vi "DSCServer.vi"() -> ()   [LabVIEW 2010]
uses:
  Ctrls/ConnectStatus.ctl
  Ctrls/DeviceModel.ctl
  Drivers/ModbusServer/Serial Config.ctl
  Drivers/ModbusServer/DeviceListChannelData.ctl
  Drivers/ModbusServer/AutoChannelData.ctl
  Ctrls/ServerData.ctl
  Ctrls/DeviceInfomation.ctl
  Ctrls/ChannelData.ctl
  Ctrls/ChannelType.ctl
  Ctrls/ChannelAccessType.ctl
  Drivers/ModbusServer/DeviceListModbusAddressRegister.ctl
  Drivers/ModbusServer/ModbusAddressRegister.ctl
  Drivers/ModbusServer/MonitorServer.lvlib
panel:
  out "连接状态":T1[](array[typedef])
  in  "驱动配置":enum32{"WatlowF4", "CM51", "DCP551", "DPR250"}(tab)
  in  "F4配置":enum32{"设备配置", "变量查看"}(tab)
  in  "DeviceList":T3[](array[typedef])
  in  "ConfigModbus":bool
  out "AllRegisterData":i16[][](array[numeric])
  out "DeviceList":string[](array[string])
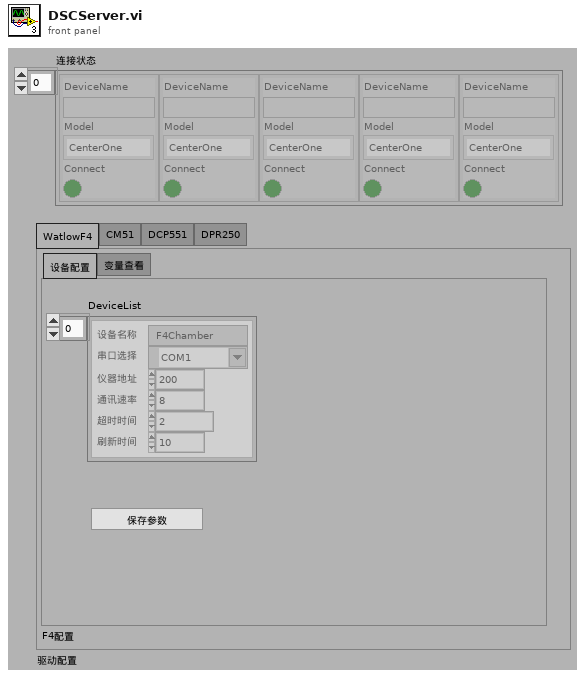
[diagram p1: front panel]
types:
  T1 = typedef "ConnectStatus.ctl" = cluster{"DeviceName":string, "Model":T2, "Connect":bool}
  T2 = typedef "DeviceModel.ctl" = enum16{"WatlowF4", "CenterOne", "DCP551", "DPR250"}
  T3 = typedef "MonitorServer.lvlib/Serial Config.ctl" = cluster{"设备名称":string, "串口选择":refnum<visa-resource-name>, "仪器地址":u32, "通讯速率":u32, "超时时间":u32, "刷新时间":dbl}
  T4 = enum32{"invalid app kind", "Development System", "Run Time System", "Student Edition", "Embedded LabVIEW", "Evaluation", "Custom"}
  T5 = enum32{"Invalid", "Standard", "Closed", "Hidden", "Minimized", "Maximized"}
  T6 = cluster{"Core":cluster{"Current VI Reference":refnum<vi>, "Close Panel on Exit?":bool}, "Your Boolean data":bool, "Your string data":string}
  T7 = cluster{"Current VI Reference":refnum<vi>, "Close Panel on Exit?":bool}
  T8 = typedef "MonitorServer.lvlib/DeviceListChannelData.ctl" = T9[]
  T9 = typedef "MonitorServer.lvlib/AutoChannelData.ctl" = cluster{"DeviceName":string, "Channel1":dbl, "SetPoint1":dbl, "Channel2":dbl, "SetPoint2":dbl, "ConnectOK":bool, "DecimalPoint1":i16, "DecimalPoint2":i16}
  T10 = typedef "MonitorServer.lvlib/DeviceListModbusAddressRegister.ctl" = T11[]
  T11 = typedef "MonitorServer.lvlib/ModbusAddressRegister.ctl" = cluster{"DeviceName":string, "AllRegisterData":i16[]}
  T12 = typedef "ServerData.ctl" = T13[]
  T13 = typedef "DeviceInfomation.ctl" = cluster{"Model":T2, "ChamberName":string, "ChannelNumber":i32, "ChannelsData":T14[], "Connected":bool}
  T14 = typedef "ChannelData.ctl" = cluster{"ChannelName":string, "ChannelType":T15, "AccessType":T16, "ProcessValue":dbl, "SetValue":dbl, "NewSettValue":dbl, "SetNewTarget":bool}
  T15 = typedef "ChannelType.ctl" = enum16{"Temperature", "Humidity"}
  T16 = typedef "ChannelAccessType.ctl" = enum16{"ReadOnly", "SetTarget"}
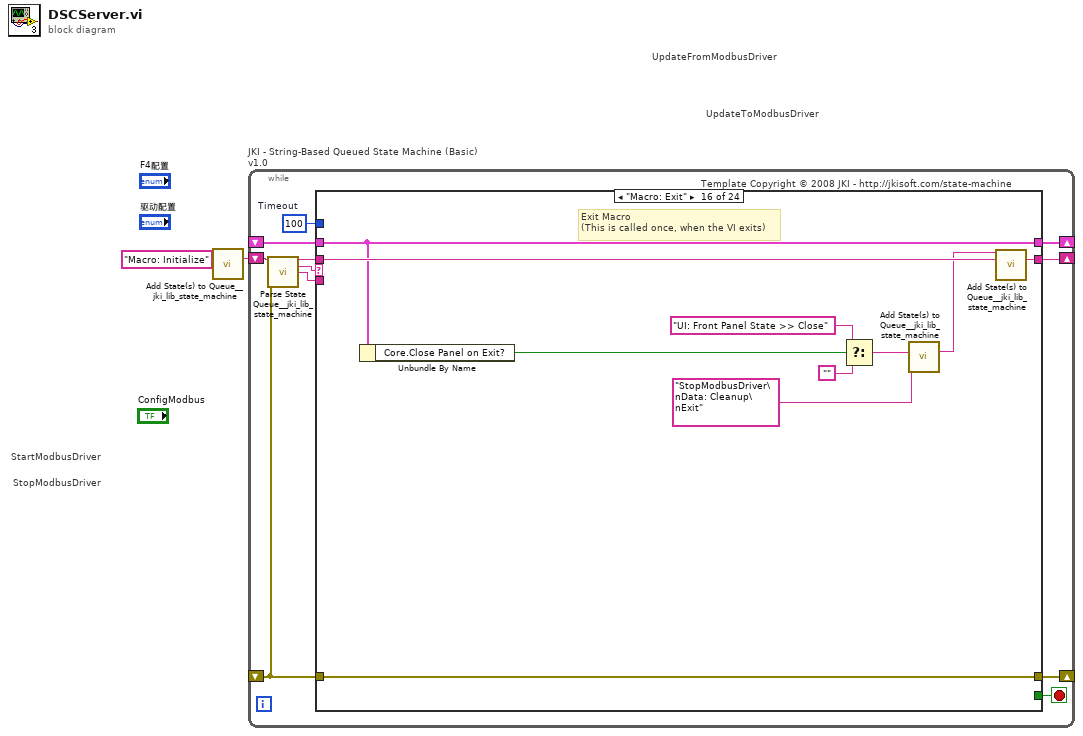
[diagram p0: block diagram]
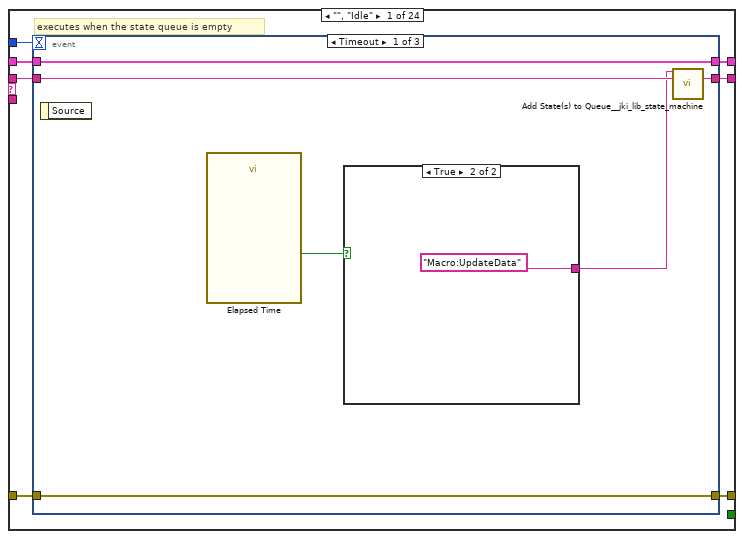
[diagram p2: hidden frame]
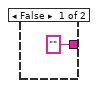
[diagram p3: hidden frame]
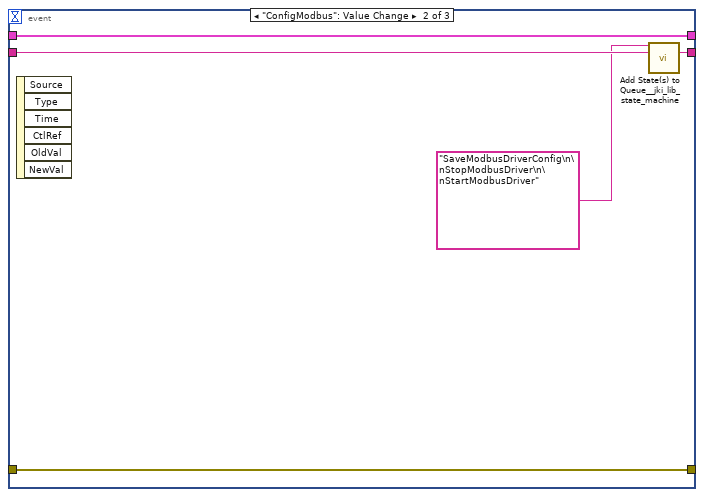
[diagram p4: hidden frame]
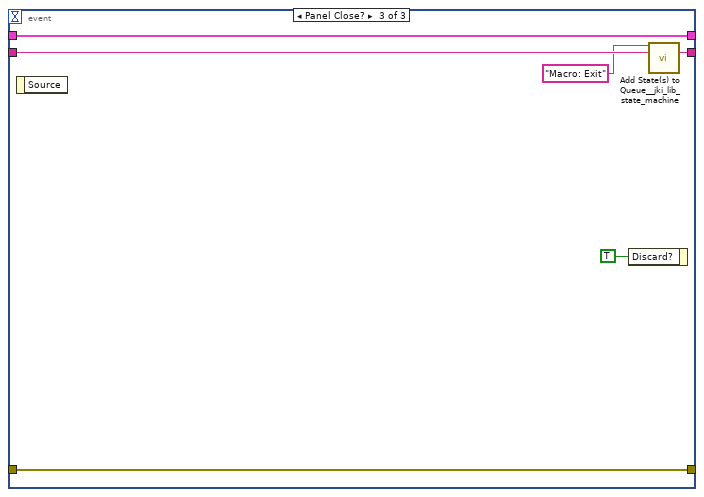
[diagram p5: hidden frame]
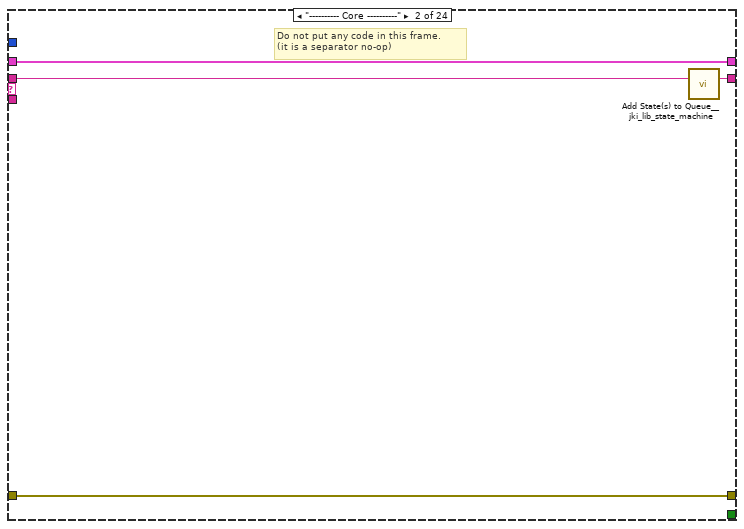
[diagram p6: hidden frame]
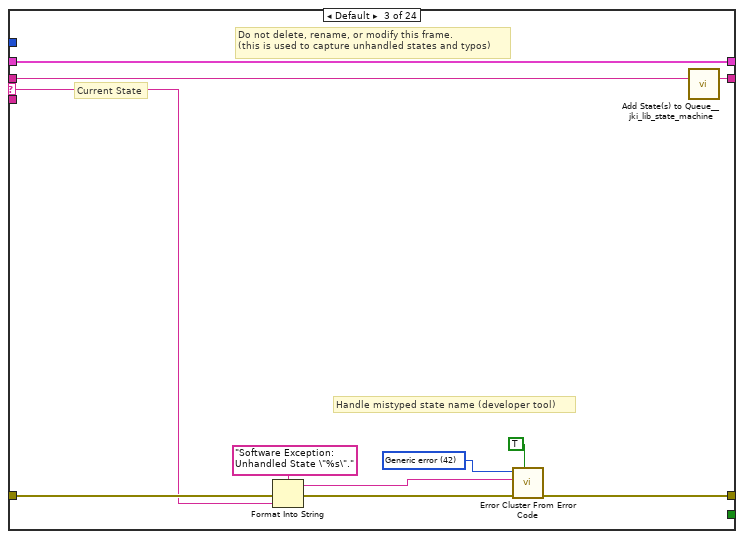
[diagram p7: hidden frame]
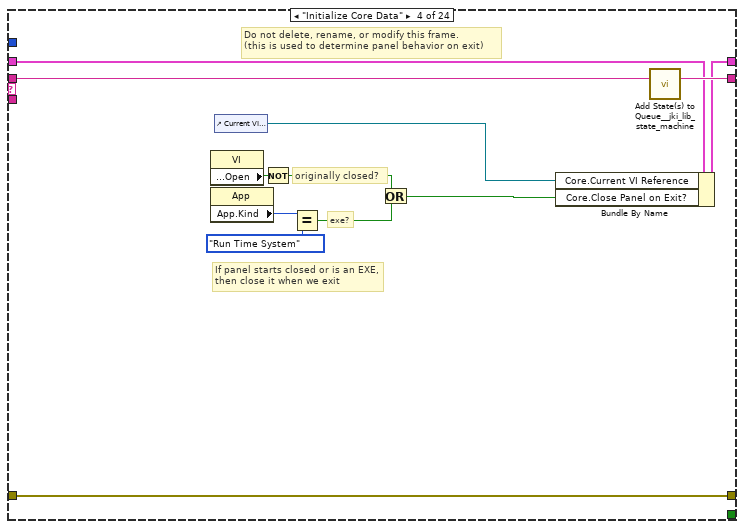
[diagram p8: hidden frame]
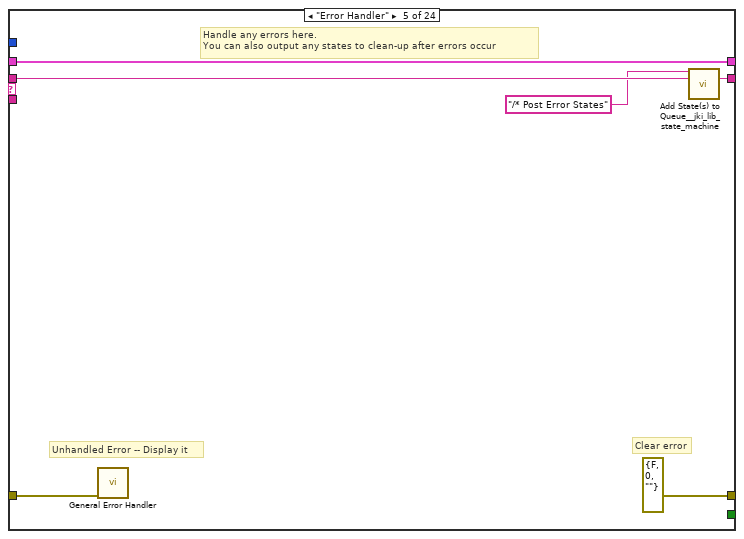
[diagram p9: hidden frame]
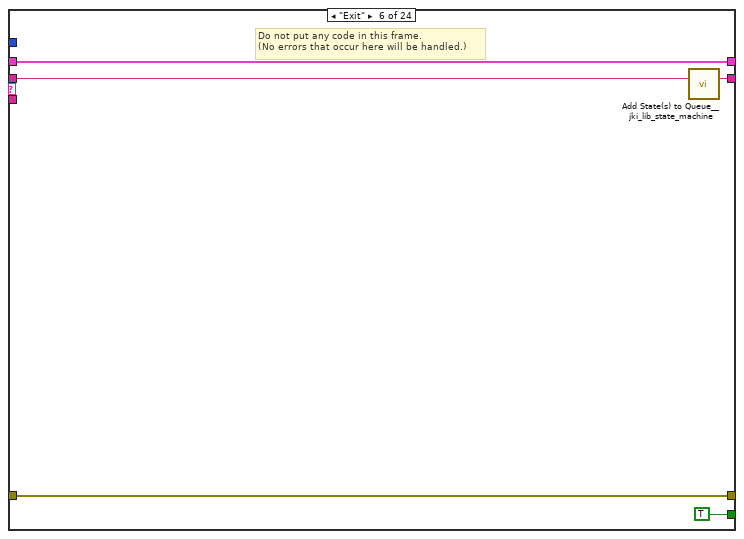
[diagram p10: hidden frame]
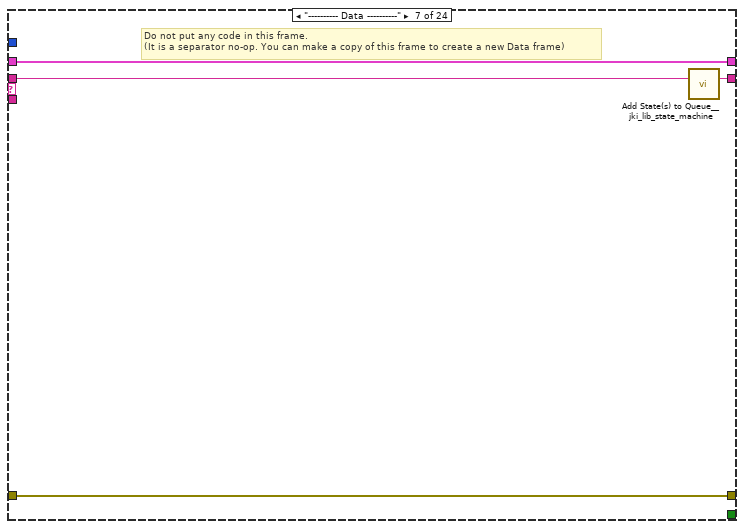
[diagram p11: hidden frame]
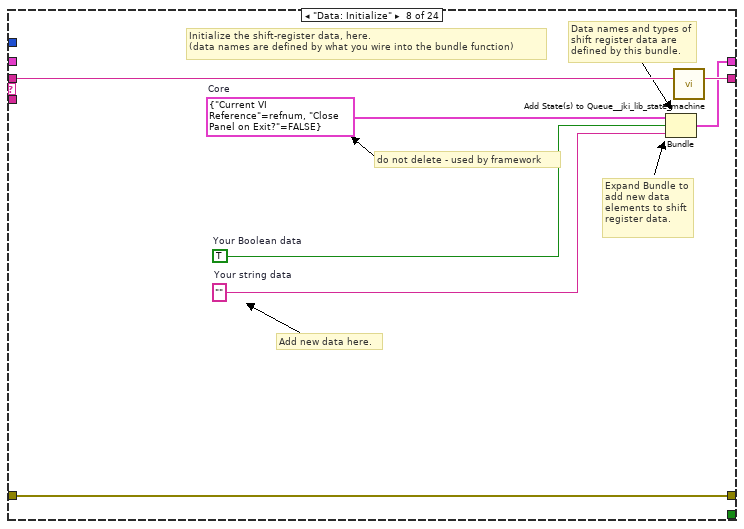
[diagram p12: hidden frame]
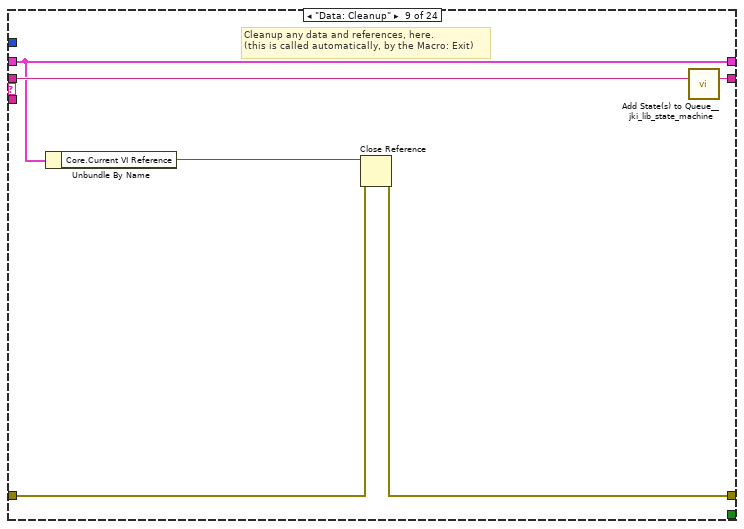
[diagram p13: hidden frame]
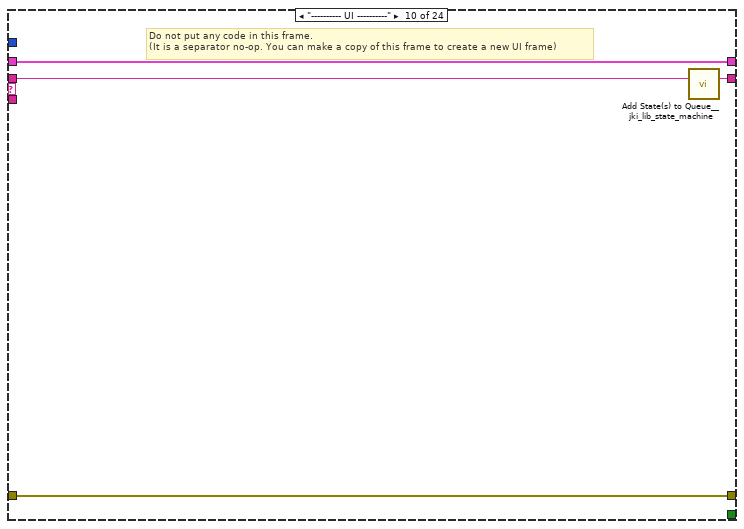
[diagram p14: hidden frame]
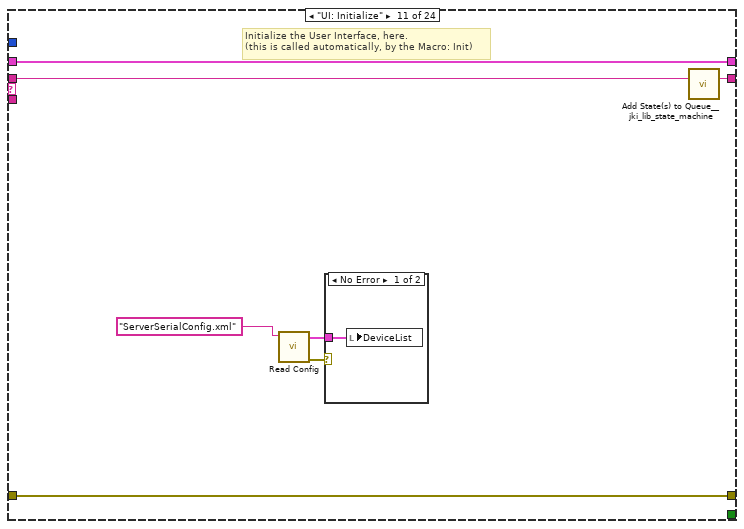
[diagram p15: hidden frame]
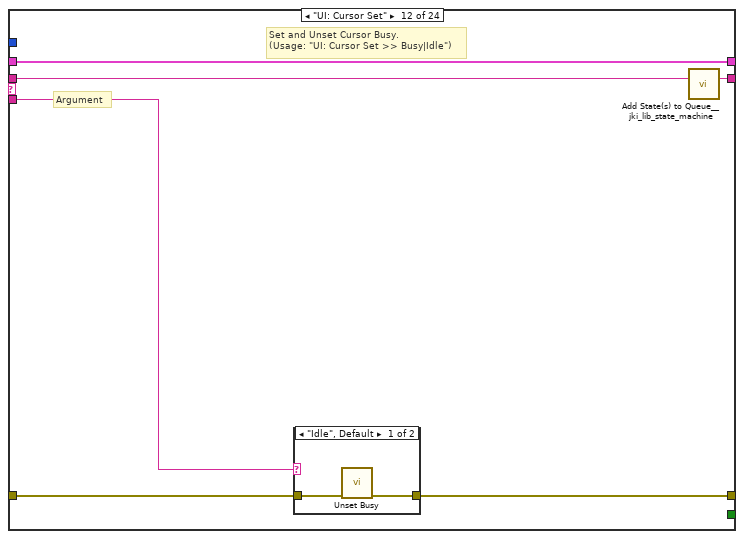
[diagram p17: hidden frame]
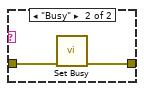
[diagram p18: hidden frame]
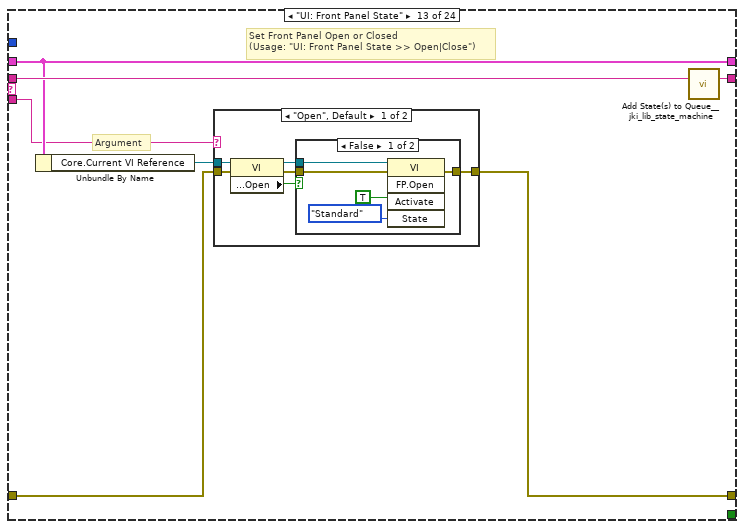
[diagram p19: hidden frame]
diagram:
  # "StopModbusDriver"
  # "StartModbusDriver"
  # "UpdateToModbusDriver"
  # "UpdateFromModbusDriver"
  n1 = call "Add State(s) to Queue__jki_lib_state_machine.vi"("State(s) in (\"\")"="Macro: Initialize") -> ("States Out"=w1:string)  [unwired: 14 in]
  n2 = while "JKI - String-Based Queued State Machine (Basic) v1.0" {
    shift-right: [w6] -> _
    shift-left: _ -> [w5]
    shift-right: [w9] -> _
    shift-left: _ -> [w3]
    shift-right: [w8] -> _
    shift-left: w1 -> [w10]
    stop <- w7 stop-if-true
    w4 = 100  # Timeout
    # "Template Copyright © 2008 JKI - http://jkisoft.com/state-machine"
    n3 = call "Parse State Queue__jki_lib_state_machine.vi"("State Queue"=w10, "Error In (no error)"=w3) -> ("Remaining States"=w12:string, "Current State"=w13:string, "Arguments"=w11:string)  [unwired: 11 in]
    n4 = case shown="\"Macro: Exit\"" w13 {
      selector: w13 -> [_ _ w44 _ _ _ _ _ _ _ _ _ _ _ _ _ _ _ _ _ _ _ _ _]
      tunnel: w12 -> [w20 w43 w48 w66 w72 w77 w81 w88 w94 w98 w105 w112 w123 w149 w154 w164 w169 w173 w179 w183 w187 w197 w206 w210]
      tunnel: w11 -> [_ _ _ _ _ _ _ _ _ _ _ w107 w117 _ _ _ _ _ _ _ _ _ _ _]
      tunnel: w5 -> [w18 w40 w46 w57 w69 w75 w78 _ w89 w95 w103 w110 w119 w146 w151 w161 w166 w170 w176 w180 w184 w194 w203 w207]
      tunnel: [w17 w41 w50 w63 errorcluster {"status"=FALSE, "code"=0, "source"=""} ("error out") w74 w79 w85 w90 w96 w102 w108 w120 w147 w152 w162 w167 w171 w177 w181 w185 w195 w204 w208] -> w9
      tunnel: w3 -> [w16 w41 w49 w63 w68 w74 w79 w85 w91 w96 w102 w109 w121 w147 w152 w162 w167 w171 w177 w181 w185 w195 w204 w208]
      tunnel: [w19 w42 w47 w65 w71 w76 w80 w87 w93 w97 w104 w111 w122 w148 w153 w163 w168 w172 w178 w182 w186 w196 w205 w209] -> w8
      tunnel: [_ _ _ _ _ TRUE _ _ _ _ _ _ _ _ _ _ _ _ _ _ _ _ _ _] -> w7
      tunnel: [w15 w40 w46 w64 w69 w75 w78 w86 w89 w95 w103 w110 w119 w146 w151 w161 w166 w170 w176 w180 w184 w194 w203 w207] -> w6
      tunnel: w4 -> [w14 _ _ _ _ _ _ _ _ _ _ _ _ _ _ _ _ _ _ _ _ _ _ _]
      frame "", "Idle" {
        # "executes when the state queue is empty"
        n5 = event shown="[0] Timeout" {
          selector: _ -> [_ _ _]
          dyn-events: _ -> [_ _ _]
          timeout: w14 -> [_ _ _]
          tunnel: w20 -> [w26 w33 w39]
          tunnel: [w25 w32 w38] -> w19
          tunnel: w18 -> [w23 w30 w36]
          tunnel: [w24 w31 w37] -> w17
          tunnel: w16 -> [w24 w31 w37]
          tunnel: [w23 w30 w36] -> w15
          event Timeout {
            n6 = event-data() -> ()  [unwired: 1 in, 1 out]
            n7 = call "Elapsed Time"() -> ("Time has Elapsed"=w22:bool)  [unwired: 12 in, 7 out]
            n8 = case shown="True" w22 {
              tunnel: ["" ("State(s) in Front (\"\")") "Macro:UpdateData" ("State(s) in Front (\"\")")] -> w21
              frame False {
              }
              frame True {
              }
            }
            n9 = call "Add State(s) to Queue__jki_lib_state_machine.vi"("State(s) in Front (\"\")"=w21, "State(s) in (\"\")"=w26) -> ("States Out"=w25:string)  [unwired: 13 in]
          }
          event "ConfigModbus": Value Change {
            n10 = event-data() -> ()  [unwired: 1 in, 6 out]
            n11 = call "Add State(s) to Queue__jki_lib_state_machine.vi"("State(s) in Front (\"\")"="SaveModbusDriverConfig\n\nStopModbusDriver\n\nStartModbusDriver" ("State(s) in Front (\"\")"), "State(s) in (\"\")"=w33) -> ("States Out"=w32:string)  [unwired: 13 in]
          }
          event Panel Close? {
            n12 = event-data() -> ()  [unwired: 1 in, 1 out]
            n13 = event-data("Discard?"=TRUE) -> ()  [unwired: 1 in, 1 out]
            n14 = call "Add State(s) to Queue__jki_lib_state_machine.vi"("State(s) in Front (\"\")"="Macro: Exit", "State(s) in (\"\")"=w39) -> ("States Out"=w38:string)  [unwired: 13 in]
          }
        }
      }
      frame "---------- Core ----------" {
        # "Do not put any code in this frame.\n(it is a separator no-op)"
        n15 = call "Add State(s) to Queue__jki_lib_state_machine.vi"("State(s) in (\"\")"=w43) -> ("States Out"=w42:string)  [unwired: 14 in]
      }
      frame Default {
        w53 = 42 items=["No error", "Argument error", "Memory is full", "Out of zone", "End of file", "File already open", "Generic file I/O error", "File not found", "File permission error", "Disk is full", "Duplicate path", "Too many files open", "System feature not enabled", "Resource file not found", "Cannot add resource", "Resource not found", "Image not found", "Image memory error", "Pen does not exist", "Config type invalid", "Config token not found", "Config parse error", "Config memory error", "Bad external code format", "Bad external code offset", "External code not present", "Null window", "Destroy window error", "Null menu", "Print aborted", "Bad print record", "Print driver error", "Windows error during printing", "Memory error during printing", "Print dialog error", "Generic print error", "Invalid device refnum", "Device not found", "Device parameter error", "Device unit error", "Cannot open device", "Device call aborted", "Generic error", "Cancelled by user", "Object ID too low", "Object ID too high", "Object not in heap", "Unknown heap", "Unknown object (invalid DefProc)", "Unknown object (DefProc not in table)", "Message out of range", "Invalid (null) method", "Unknown message", "Manager call not supported", "Bad address", "Network operation in progress", "Network operation timed out", "Connection is busy", "Network attribute not supported", "Network error", "Address in use", "System out of memory", "Connection aborted", "Connection refused", "Not connected", "Already connected", "Connection closed", "Initialization error (interapplication manager)", "Bad occurrence", "Wait on unbound occurrence handler", "Occurrence queue overflow", "Datalog type conflict", "Unused", "Unrecognized type (interapplication manager)", "Memory corrupt", "Failed to make temporary DLL", "Old CIN version", "Drag socket not found", "Failed to load drop-object", "Failed to register OLE object", "Failed to release OLE object", "Format specifier type mismatch", "Unknown format specifier", "Too few format specifiers", "Too many format specifiers", "Scan failed", "Newer CIN version", "Error converting to variant", "Runtime menu error", "Password tampered", "Variant attribute not found", "Incompatible variant data type", "Event data is not available", "Event Store is not present", "Occurrence is not found", "Event Queue is not created", "Event info is not available", "Refnum passed is NULL", "Error retrieving Class GUID", "Error retrieving CoClass GUID", "Error retrieving TypeLib GUID.", "Bad built application magic bytes.", "Specific driver is different from the specific driver associated with the Logical Name.", "There is no session opened to the class driver.", "Max Error", "MAX - Error with config objects", "MAX - Error loading configuration", "MAX - Group not supported"]
        # "Current State"
        # "Do not delete, rename, or modify this frame.\n(this is used to capture unhandled states and typos)"
        # "Handle mistyped state name (developer tool)"
        n16 = Format Into String(format string="Software Exception: Unhandled State \"%s\"." ("message"), error in=w49, w44) -> (resulting string=w52:string, error out=w51:errorcluster)  [unwired: 1 in]
        n17 = call <vilib>:"Error Cluster From Error Code.vi"("show call chain? (False)"=TRUE, "error in (no error)"=w51, "error message (\"\")"=w52, "error code (0)"=w53) -> ("error out"=w50:errorcluster)  [unwired: 5 in]
        n18 = call "Add State(s) to Queue__jki_lib_state_machine.vi"("State(s) in (\"\")"=w48) -> ("States Out"=w47:string)  [unwired: 14 in]
      }
      frame "Initialize Core Data" {
        # "Do not delete, rename, or modify this frame.\n(this is used to determine panel behavior on exit)"
        # "originally closed?"
        # "exe?"
        # "If panel starts closed or is an EXE, then close it when we exit"
        n19 = property class="VI"() -> ("Front Panel.Open"=w62:bool)  [unwired: 2 in, 2 out]
        n20 = property class="App"() -> ("App.Kind"=w61:T4)  [unwired: 2 in, 2 out]
        n21 = control-ref of="Current VI Reference"() -> (w55:refnum<vi>)
        n22 = Not(x=w62) -> (.not. x?=w59:bool)
        n23 = Equal?(x=w61, y=T4."Run Time System" ("Application:Kind")) -> (x = y?=w58:bool)
        n24 = Or(x=w59, y=w58) -> (x .or. y?=w56:bool)
        n25 = Bundle By Name(cluster=w57, "Core.Current VI Reference"=w55, "Core.Close Panel on Exit?"=w56) -> (w64:T6)
        n26 = call "Add State(s) to Queue__jki_lib_state_machine.vi"("State(s) in (\"\")"=w66) -> ("States Out"=w65:string)  [unwired: 14 in]
      }
      frame "Error Handler" {
        # "Unhandled Error -- Display it"
        # "Handle any errors here.\nYou can also output any states to clean-up after errors occur"
        # "Clear error"
        n27 = call <vilib>:"General Error Handler.vi"("error in (no error)"=w68) -> ()  [unwired: 10 in, 5 out]
        n28 = call "Add State(s) to Queue__jki_lib_state_machine.vi"("State(s) in Front (\"\")"="/* Post Error States", "State(s) in (\"\")"=w72) -> ("States Out"=w71:string)  [unwired: 13 in]
      }
      frame "Exit" {
        # "Do not put any code in this frame.\n(No errors that occur here will be handled.)"
        n29 = call "Add State(s) to Queue__jki_lib_state_machine.vi"("State(s) in (\"\")"=w77) -> ("States Out"=w76:string)  [unwired: 14 in]
      }
      frame "---------- Data ----------" {
        # "Do not put any code in this frame.\n(It is a separator no-op. You can make a copy of this frame to create a new Data frame)"
        n30 = call "Add State(s) to Queue__jki_lib_state_machine.vi"("State(s) in (\"\")"=w81) -> ("States Out"=w80:string)  [unwired: 14 in]
      }
      frame "Data: Initialize" {
        w82 = T7 {"Current VI Reference"=refnum, "Close Panel on Exit?"=FALSE}  # Core
        w84 = TRUE  # Your Boolean data
        w83 = ""  # Your string data
        # "do not delete - used by framework"
        # "Expand Bundle to add new data elements to shift register data."
        # "Add new data here."
        # "Data names and types of shift register data are defined by this bundle."
        # "Initialize the shift-register data, here.\n(data names are defined by what you wire into the bundle function)"
        n31 = Bundle("Core"=w82, "Your Boolean data"=w84, "Your string data"=w83) -> (w86:T6)  [unwired: 1 in]
        n32 = call "Add State(s) to Queue__jki_lib_state_machine.vi"("State(s) in (\"\")"=w88) -> ("States Out"=w87:string)  [unwired: 14 in]
      }
      frame "Data: Cleanup" {
        # "Cleanup any data and references, here.\n(this is called automatically, by the Macro: Exit)"
        n33 = Unbundle By Name(w89) -> ("Core.Current VI Reference"=w92:refnum<vi>)
        n34 = Close Reference(reference=w92, error in (no error)=w91) -> (error out=w90:errorcluster)
        n35 = call "Add State(s) to Queue__jki_lib_state_machine.vi"("State(s) in (\"\")"=w94) -> ("States Out"=w93:string)  [unwired: 14 in]
      }
      frame "---------- UI ----------" {
        # "Do not put any code in this frame.\n(It is a separator no-op. You can make a copy of this frame to create a new UI frame)"
        n36 = call "Add State(s) to Queue__jki_lib_state_machine.vi"("State(s) in (\"\")"=w98) -> ("States Out"=w97:string)  [unwired: 14 in]
      }
      frame "UI: Initialize" {
        # "Initialize the User Interface, here.\n(this is called automatically, by the Macro: Init)"
        n37 = call "Read Config.vi"("ConfigurationFileName"="ServerSerialConfig.xml" ("FileName")) -> ("error out"=w99:errorcluster, "DeviceList"=w100:T3[])  [unwired: 9 in]
        n38 = case shown="No Error" w99 {
          tunnel: w100 -> [w106 _]
          frame No Error {
            n39 = local write "DeviceList"(w106) -> ()
          }
          frame Error {
          }
        }
        n40 = call "Add State(s) to Queue__jki_lib_state_machine.vi"("State(s) in (\"\")"=w105) -> ("States Out"=w104:string)  [unwired: 14 in]
      }
      frame "UI: Cursor Set" {
        # "Argument"
        # "Set and Unset Cursor Busy.\n(Usage: \"UI: Cursor Set >> Busy|Idle\")"
        n41 = case shown="\"Idle\", Default" w107 {
          tunnel: w109 -> [w114 w116]
          tunnel: [w113 w115] -> w108
          frame "Idle", Default {
            n42 = call <vilib>:"Unset Busy.vi"("error in (no error)"=w114) -> ("error out"=w113:errorcluster)  [unwired: 10 in]
          }
          frame "Busy" {
            n43 = call <vilib>:"Set Busy.vi"("error in (no error)"=w116) -> ("error out"=w115:errorcluster)  [unwired: 9 in, 1 out]
          }
        }
        n44 = call "Add State(s) to Queue__jki_lib_state_machine.vi"("State(s) in (\"\")"=w112) -> ("States Out"=w111:string)  [unwired: 14 in]
      }
      frame "UI: Front Panel State" {
        # "Argument"
        # "Set Front Panel Open or Closed\n(Usage: \"UI: Front Panel State >> Open|Close\")"
        n45 = Unbundle By Name(w119) -> ("Core.Current VI Reference"=w118:refnum<vi>)
        n46 = case shown="\"Open\", Default" w117 {
          tunnel: w121 -> [w127 w140]
          tunnel: [w129 w141] -> w120
          tunnel: w118 -> [w128 w138]
          frame "Open", Default {
            n47 = property class="VI"(reference=w128, error in=w127) -> (reference out=w125:refnum<vi>, error out=w126:errorcluster, "Front Panel.Open"=w124:bool)
            n48 = case shown="False" w124 {
              tunnel: [w132 w135] -> w129
              tunnel: w126 -> [w131 w135]
              tunnel: w125 -> [w130 _]
              frame False {
                n49 = invoke class="VI" method="FP.Open"(reference=w130, error in=w131, "Activate"=TRUE, "State"=T5."Standard") -> (error out=w132:errorcluster)  [unwired: 1 in, 4 out]
              }
              frame True {
              }
            }
          }
          frame "Close" {
            n50 = property class="VI"(reference=w138, error in=w140) -> (reference out=w137:refnum<vi>, error out=w139:errorcluster, "Front Panel.Open"=w136:bool)
            n51 = case shown="True" w136 {
              tunnel: [w142 w145] -> w141
              tunnel: w139 -> [w142 w144]
              tunnel: w137 -> [_ w143]
              frame False {
              }
              frame True {
                n52 = invoke class="VI" method="FP.Close"(reference=w143, error in=w144) -> (error out=w145:errorcluster)  [unwired: 1 in, 2 out]
              }
            }
          }
        }
        n53 = call "Add State(s) to Queue__jki_lib_state_machine.vi"("State(s) in (\"\")"=w123) -> ("States Out"=w122:string)  [unwired: 14 in]
      }
      frame "---------- Macro ----------" {
        # "Do not put any code in this frame.\n(It is a separator no-op. You can make a copy of this frame to create a new Macro frame)"
        n54 = call "Add State(s) to Queue__jki_lib_state_machine.vi"("State(s) in (\"\")"=w149) -> ("States Out"=w148:string)  [unwired: 14 in]
      }
      frame "Macro: Initialize" {
        w150 = "Data: Initialize\nInitialize Core Data\nUI: Initialize\nUI: Front Panel State >> Open\nStartModbusDriver\n"  # Data: Initialize Initialize Core Data UI: Initialize UI: Front Panel State >> Open StartModbusDriver
        # "Initialization Macro\n(This is called once, when the VI starts)"
        n55 = call "Add State(s) to Queue__jki_lib_state_machine.vi"("State(s) in Front (\"\")"=w150, "State(s) in (\"\")"=w154) -> ("States Out"=w153:string)  [unwired: 13 in]
      }
      frame "Macro: Exit" {
        # "Exit Macro\n(This is called once, when the VI exits)"
        n56 = Unbundle By Name(w161) -> ("Core.Close Panel on Exit?"=w160:bool)
        n57 = Select(t="UI: Front Panel State >> Close", s=w160, f="") -> (s? t:f=w157:string)
        n58 = call "Add State(s) to Queue__jki_lib_state_machine.vi"("State(s) in (\"\")"=w157, "State(s) at Back (\"\")"="StopModbusDriver\nData: Cleanup\nExit") -> ("States Out"=w155:string)  [unwired: 13 in]
        n59 = call "Add State(s) to Queue__jki_lib_state_machine.vi"("State(s) in Front (\"\")"=w155, "State(s) in (\"\")"=w164) -> ("States Out"=w163:string)  [unwired: 13 in]
      }
      frame "Macro:UpdateData" {
        # "Exit Macro\n(This is called once, when the VI exits)"
        n60 = call "Add State(s) to Queue__jki_lib_state_machine.vi"("State(s) in Front (\"\")"="UpdateFromModbusDriver\nUpdateToModbusDriver" ("State(s) in Front (\"\")"), "State(s) in (\"\")"=w169) -> ("States Out"=w168:string)  [unwired: 13 in]
      }
      frame "---------- ModbusDriver ----------" {
        # "Template Separator\n(You can make a copy of, or modify, this frame)"
        n61 = call "Add State(s) to Queue__jki_lib_state_machine.vi"("State(s) in (\"\")"=w173) -> ("States Out"=w172:string)  [unwired: 14 in]
      }
      frame "SaveModbusDriverConfig" {
        # "Your code here.\n(You can make a copy of, or modify, this frame)"
        n62 = call "Save Config.vi"("FileName"="ServerSerialConfig.xml", "DeviceList"="DeviceList") -> ()  [unwired: 9 in, 1 out]
        n63 = call "Add State(s) to Queue__jki_lib_state_machine.vi"("State(s) in (\"\")"=w179) -> ("States Out"=w178:string)  [unwired: 14 in]
      }
      frame "StartModbusDriver" {
        # "Your code here.\n(You can make a copy of, or modify, this frame)"
        n64 = call "StartServer.vi"() -> ()  [unwired: 11 in, 1 out]
        n65 = call "Add State(s) to Queue__jki_lib_state_machine.vi"("State(s) in (\"\")"=w183) -> ("States Out"=w182:string)  [unwired: 14 in]
      }
      frame "StopModbusDriver" {
        # "Your code here.\n(You can make a copy of, or modify, this frame)"
        n66 = call "StopServer.vi"() -> ()  [unwired: 11 in, 1 out]
        n67 = call "Add State(s) to Queue__jki_lib_state_machine.vi"("State(s) in (\"\")"=w187) -> ("States Out"=w186:string)  [unwired: 14 in]
      }
      frame "UpdateFromModbusDriver" {
        n68 = shared-variable "My Computer\\MonitorServer.lvlib\\AutoReadChannels"() -> (w193:T8)  [unwired: 1 in, 1 out]
        n69 = shared-variable "My Computer\\MonitorServer.lvlib\\DeviceListRegister"() -> (w190:T10)  [unwired: 1 in, 1 out]
        n70 = for {
          tunnel: w190 -> [w200] mode=indexing
          tunnel: [w199] -> w188 mode=indexing
          tunnel: [w198] -> w189 mode=indexing
          n71 = Unbundle By Name(w200) -> ("DeviceName"=w199:string, "AllRegisterData"=w198:i16[])
        }
        "AllRegisterData" <- w189
        "DeviceList" <- w188
        n72 = call "ModbusDriverDataToServer.vi"("DeviceListChannelData"=w193) -> ("ServerData"=w192:T12, "Status"=→"连接状态":T1[])  [unwired: 9 in]
        n73 = shared-variable "My Computer\\DSCServer.lvlib\\ServerData"(w192) -> ()  [unwired: 1 in, 1 out]
        n74 = call "Add State(s) to Queue__jki_lib_state_machine.vi"("State(s) in (\"\")"=w197) -> ("States Out"=w196:string)  [unwired: 14 in]
      }
      frame "UpdateToModbusDriver" {
        n75 = shared-variable "My Computer\\MonitorServer.lvlib\\AutoReadChannels"() -> (w201:T8)  [unwired: 1 in, 1 out]
        n76 = shared-variable "My Computer\\DSCServer.lvlib\\ServerData"() -> (w202:T12)  [unwired: 1 in, 1 out]
        n77 = call "SetTarget.vi"("AutoReadChannels"=w201, "ServerData"=w202) -> ()  [unwired: 10 in]
        n78 = call "Add State(s) to Queue__jki_lib_state_machine.vi"("State(s) in (\"\")"=w206) -> ("States Out"=w205:string)  [unwired: 14 in]
      }
      frame "---------- Server ----------" {
        # "Template Separator\n(You can make a copy of, or modify, this frame)"
        n79 = call "Add State(s) to Queue__jki_lib_state_machine.vi"("State(s) in (\"\")"=w210) -> ("States Out"=w209:string)  [unwired: 14 in]
      }
    }
  }
